vi "Filtr(SubVI).vi"(2 "Dolni Mezni Frekvence":dbl=0.125 format="%0.2f", 3 "Horni Mezni Frekvence":dbl=0.45 format="%0.2f", 4 "Typ Filtru":T1, 5 "Vstupni Waveform":waveform(dbl)) -> (0 "Spektrum":cluster{"f0":dbl, "df":dbl, "magnitude":dbl[]} {"magnitude" format="%.2p"; "f0" format="%0.2p"; "df" format="%0.2p"}, 1 "Vystupni Waveform":waveform(dbl))   [LabVIEW 2025]
uses:
  <vilib>/Analysis/3filter.llb/Filter Passband Type.ctl
  <vilib>/Analysis/3filter.llb/FIR Windowed Filter (DBL).vi
  <vilib>/Analysis/NI_AALBase.lvlib
  <vilib>/measure/NI_MAPro.lvlib
  <vilib>/measure/maspectr.llb/FFT Spectrum (Mag-Phase) for 1 Chan.vi
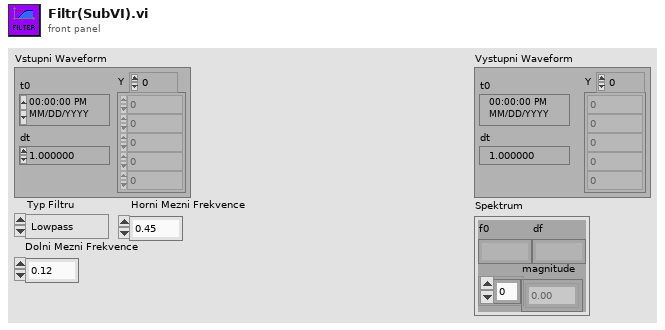
[diagram p1: front panel]
types:
  T1 = typedef "NI_AALBase.lvlib/Filter Passband Type.ctl" = enum32{"Lowpass", "Highpass", "Bandpass", "Bandstop"}
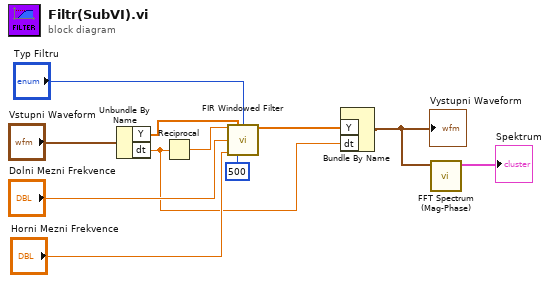
[diagram p0: block diagram]
diagram:
  n1 = Unbundle By Name("Vstupni Waveform") -> ("Y"=w10:dbl[], "dt"=w3:dbl)
  n2 = Reciprocal(x=w3) -> (1/x=w11:dbl)
  n3 = call-poly <vilib>:"FIR Windowed Filter.vi"("sampling freq: fs"=w11, "X"=w10, "filter type"="Typ Filtru", "low cutoff freq: fl"="Dolni Mezni Frekvence", "high cutoff freq: fh"="Horni Mezni Frekvence", "taps"=500) -> ("Filtered X"=w5:dbl[])  [unwired: 8 in, 1 out]
  n4 = Bundle By Name("Y"=w5, "dt"=w3) -> (w2:waveform(dbl))  [unwired: 1 in]
  "Vystupni Waveform" <- w2
  n5 = call-poly <vilib>:"FFT Spectrum (Mag-Phase).vi"("time signal"=w2) -> ("magnitude"=→"Spektrum":cluster{"f0":dbl, "df":dbl, "magnitude":dbl[]})  [unwired: 6 in, 4 out]
